vi "BuildDataLogical.vi"(9 "new element/subarray":bool, 11 "element":bool) -> (2 "[0]":bool)   [LabVIEW 2011]
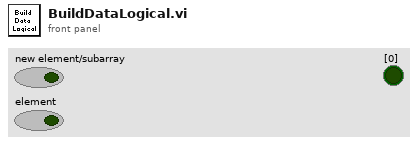
[diagram p1: front panel]
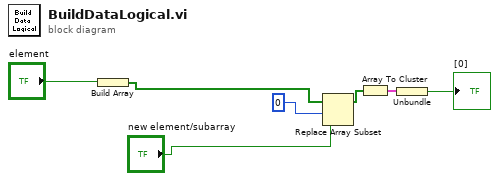
[diagram p0: block diagram]
diagram:
  n1 = Build Array("element") -> (w7:bool[])
  n2 = Replace Array Subset(array=w7, new element="new element/subarray", index=0) -> (w4:bool[])
  n3 = Array To Cluster(array=w4) -> (cluster=w6:cluster{"[0]":bool})
  n4 = Unbundle(w6) -> ("[0]"=→"[0]":bool)
